vi "Test - Quick Invert.vi"() -> ()   [LabVIEW 2020, in "3D (FPGA).lvlib"]
uses:
  3D (FPGA).lvlib
panel:
  out "Point At Matrix":sgl[][](array[numeric])
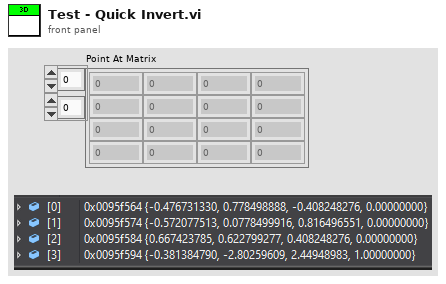
[diagram p1: front panel]
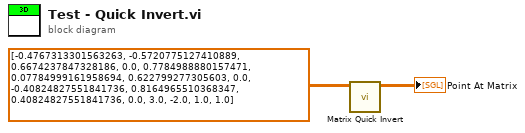
[diagram p0: block diagram]
diagram:
  n1 = call "Matrix Quick Invert.vi"("Matrix"=sgl[][] [[-0.47673133, -0.5720775, 0.6674238, 0.0], [0.7784989, 0.07784999, 0.6227993, 0.0], [-0.40824828, 0.81649655, 0.40824828, 0.0], [3.0, -2.0, 1.0, 1.0]] ("Point At Matrix")) -> ("Matrix Inverted"=→"Point At Matrix":sgl[][])  [unwired: 10 in]
